vi "Get Possible Unit Conversions.vi"(1 "Quantity":T1, 2 "Base Unit":T2) -> (0 "Possible Target Units":T2[](array[typedef]))   [LabVIEW 2023, in "NI_HFNetworkAnalysis.lvlib"]
doc: "Retrieve the possible unit conversion for the specified quantity expressed in the base unit."
uses:
  NI_HFNetworkAnalysis.lvlib
  Controls/Unit.ctl
  Controls/Quantity.ctl
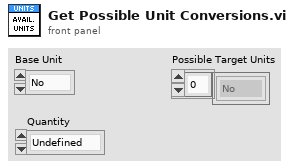
[diagram p1: front panel]
types:
  T1 = typedef "NI_HFNetworkAnalysis.lvlib/Quantity.ctl" = enum16{"Undefined", "V", "I", "A", "B", "P", "Z", "PowerRatio", "Gamma", "Index"}
  T2 = typedef "NI_HFNetworkAnalysis.lvlib/Unit.ctl" = enum16{"No", "s", "Hz", "V", "A", "Ohm", "W", "dB", "dBV", "dBA", "dBm", "percent", "rad", "deg"}
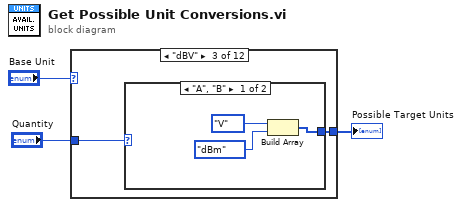
[diagram p0: block diagram]
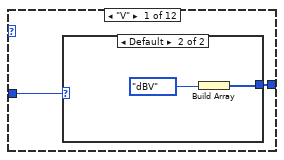
[diagram p2: hidden frame]
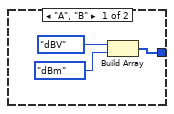
[diagram p3: hidden frame]
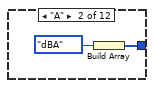
[diagram p4: hidden frame]
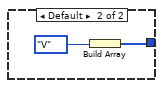
[diagram p5: hidden frame]
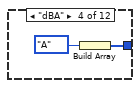
[diagram p6: hidden frame]
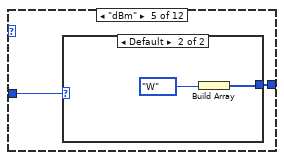
[diagram p7: hidden frame]
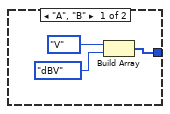
[diagram p8: hidden frame]
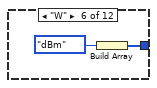
[diagram p9: hidden frame]
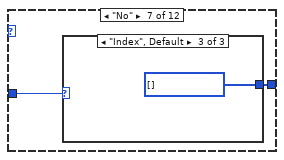
[diagram p10: hidden frame]
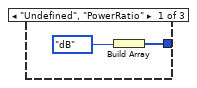
[diagram p11: hidden frame]
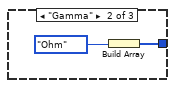
[diagram p12: hidden frame]
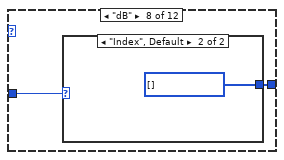
[diagram p13: hidden frame]
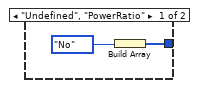
[diagram p14: hidden frame]
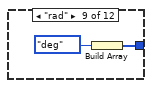
[diagram p15: hidden frame]
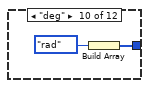
[diagram p16: hidden frame]
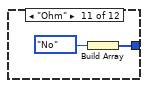
[diagram p17: hidden frame]
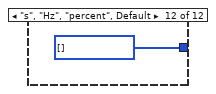
[diagram p18: hidden frame]
diagram:
  n1 = case shown="\"dBV\"" "Base Unit" {
    tunnel: "Quantity" -> [w5 _ w14 _ w23 _ w32 w39 _ _ _ _]
    tunnel: [w4 w11 w13 w20 w22 w29 w31 w38 w43 w45 w47 w49] -> w2
    frame "V" {
      n2 = case shown="Default" w5 {
        tunnel: [w8 w10] -> w4
        frame "A", "B" {
          n3 = Build Array(Unit."dBV" ("element"), Unit."dBm" ("Base Unit")) -> (w8:T2[])
        }
        frame Default {
          n4 = Build Array(Unit."dBV" ("Base Unit")) -> (w10:T2[])
        }
      }
    }
    frame "A" {
      n5 = Build Array(Unit."dBA" ("Base Unit")) -> (w11:T2[])
    }
    frame "dBV" {
      n6 = case shown="\"A\", \"B\"" w14 {
        tunnel: [w17 w19] -> w13
        frame "A", "B" {
          n7 = Build Array(Unit."V" ("element"), Unit."dBm" ("Base Unit")) -> (w17:T2[])
        }
        frame Default {
          n8 = Build Array(Unit."V" ("Base Unit")) -> (w19:T2[])
        }
      }
    }
    frame "dBA" {
      n9 = Build Array(Unit."A" ("Base Unit")) -> (w20:T2[])
    }
    frame "dBm" {
      n10 = case shown="Default" w23 {
        tunnel: [w26 w28] -> w22
        frame "A", "B" {
          n11 = Build Array(Unit."V" ("element"), Unit."dBV" ("Base Unit")) -> (w26:T2[])
        }
        frame Default {
          n12 = Build Array(Unit."W" ("Base Unit")) -> (w28:T2[])
        }
      }
    }
    frame "W" {
      n13 = Build Array(Unit."dBm" ("Base Unit")) -> (w29:T2[])
    }
    frame "No" {
      n14 = case shown="\"Index\", Default" w32 {
        tunnel: [w34 w36 w37] -> w31
        frame "Undefined", "PowerRatio" {
          n15 = Build Array(Unit."dB" ("Base Unit")) -> (w34:T2[])
        }
        frame "Gamma" {
          n16 = Build Array(Unit."Ohm" ("Base Unit")) -> (w36:T2[])
        }
        frame "Index", Default {
          w37 = T2[] [] items=["No", "s", "Hz", "V", "A", "Ohm", "W", "dB", "dBV", "dBA", "dBm", "percent", "rad", "deg"]
        }
      }
    }
    frame "dB" {
      n17 = case shown="\"Index\", Default" w39 {
        tunnel: [w41 w42] -> w38
        frame "Undefined", "PowerRatio" {
          n18 = Build Array(Unit."No" ("Base Unit")) -> (w41:T2[])
        }
        frame "Index", Default {
          w42 = T2[] [] items=["No", "s", "Hz", "V", "A", "Ohm", "W", "dB", "dBV", "dBA", "dBm", "percent", "rad", "deg"]
        }
      }
    }
    frame "rad" {
      n19 = Build Array(Unit."deg" ("Base Unit")) -> (w43:T2[])
    }
    frame "deg" {
      n20 = Build Array(Unit."rad" ("Base Unit")) -> (w45:T2[])
    }
    frame "Ohm" {
      n21 = Build Array(Unit."No" ("Base Unit")) -> (w47:T2[])
    }
    frame "s", "Hz", "percent", Default {
      w49 = T2[] [] items=["No", "s", "Hz", "V", "A", "Ohm", "W", "dB", "dBV", "dBA", "dBm", "percent", "rad", "deg"]
    }
  }
  "Possible Target Units" <- w2
